vi "Idle.vi"(8 "error in (no error)":errorcluster caption="错误输入（无错误）", 10 "iaxis":i32, 11 "handle":u32) -> (0 "error out":errorcluster caption="错误输出", 1 "Axis":i32, 2 "Speed":sgl, 3 "Dpos":sgl, 5 "State":i32)   [LabVIEW 2015]
uses:
  zauxdll-2014/zauxdll.lvlib
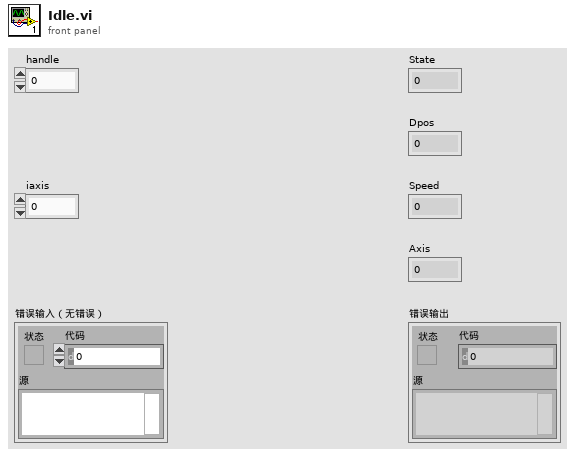
[diagram p1: front panel]
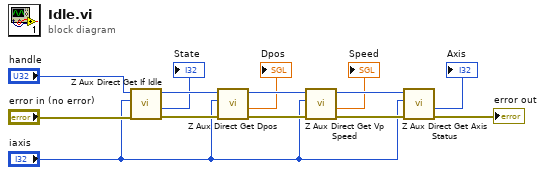
[diagram p0: block diagram]
diagram:
  n1 = call "Z Aux Direct Get If Idle.vi"("error in (no error)"="error in (no error)", "iaxis"="iaxis", "handle"="handle") -> ("error out"=w14:errorcluster, "piValue out"=→"State":i32, "handle out"=w13:u32)  [unwired: 5 in, 1 out]
  n2 = call "Z Aux Direct Get Dpos.vi"("error in (no error)"=w14, "iaxis"="iaxis", "handle"=w13) -> ("error out"=w10:errorcluster, "pfValue out"=→"Dpos":sgl, "handle out"=w12:u32)  [unwired: 5 in, 1 out]
  n3 = call "Z Aux Direct Get Vp Speed.vi"("error in (no error)"=w10, "iaxis"="iaxis", "handle"=w12) -> ("error out"=w9:errorcluster, "pfValue out"=→"Speed":sgl, "handle out"=w11:u32)  [unwired: 5 in, 1 out]
  n4 = call "Z Aux Direct Get Axis Status.vi"("error in (no error)"=w9, "iaxis"="iaxis", "handle"=w11) -> ("error out"=→"error out":errorcluster, "piValue out"=→"Axis":i32)  [unwired: 5 in, 2 out]
